vi "Manual.vi"(8 "error in":errorcluster, 10 "Manual":bool, 11 "Base Software in":refnum<class "Base Software.lvclass">) -> (0 "error out":errorcluster, 3 "Base Software out":refnum<class "Base Software.lvclass">)   [LabVIEW 2019, in "Base Software.lvlib" / "Main.lvlib" / "Base Software.lvclass"]
uses:
  Project/Base Software.lvclass
  Project/Base Software.lvclass/Base Software.ctl
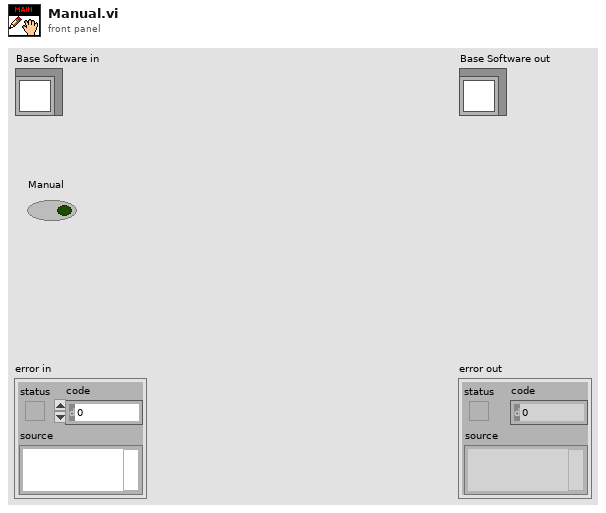
[diagram p1: front panel]
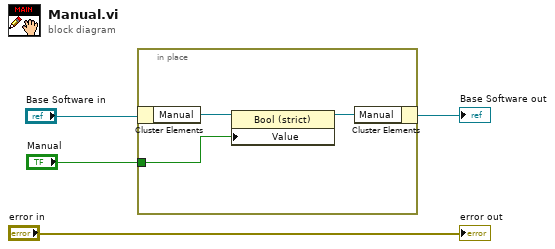
[diagram p0: block diagram]
diagram:
  n1 = in-place {
    in-place-border: "Manual" -> [w7]
    n2 = in-place-cluster #1("Base Software in") -> ("Manual"=w6:refnum<vi>)
    n3 = property class="Bool (strict)"(reference=w6, "Value"=w7) -> (reference out=w5:refnum<vi>)  [unwired: 1 in, 1 out]
    n4 = in-place-cluster #1("Manual"=w5) -> (→"Base Software out":refnum<class "Base Software.lvclass">)
  }
  "error out" <- "error in"
